vi "Write 1Ch NSamp (Timestamp).vi"(4 "timestamps":timestamp[](array[numeric]), 6 "index_channel":u32, 8 "error in":errorcluster, 9 "data":timestamp[](array[numeric]), 10 "channel":u32, 11 "Writer":refnum<class "Synnax Writer.lvclass">) -> (0 "error out":errorcluster, 3 "Writer Out":refnum<class "Synnax Writer.lvclass">)   [LabVIEW 2026, in "synnax_lib.lvlib" / "Synnax Writer.lvclass"]
uses:
  Synnax Writer.lvclass
  Synnax Writer.lvclass/Synnax Writer.ctl
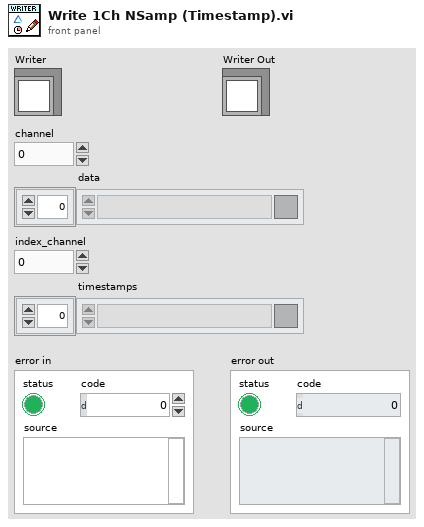
[diagram p1: front panel]
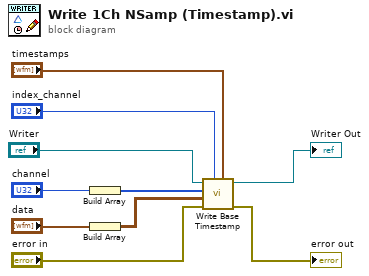
[diagram p0: block diagram]
diagram:
  n1 = Build Array("channel") -> (w7:u32[])
  n2 = Build Array("data") -> (w3:timestamp[][])
  n3 = call "Write Base Timestamp.vi"("timestamps"="timestamps", "index_channel"="index_channel", "error in"="error in", "data"=w3, "channels"=w7, "Writer"="Writer") -> ("error out"=→"error out":errorcluster, "Writer Out"=→"Writer Out":refnum<class "Synnax Writer.lvclass">)  [unwired: 4 in]
